vi "Set Configuration.vi"(10 "IConfigure":refnum<class "IConfigure.lvclass">, 11 "Instrument Factory in":refnum<class "Instrument Factory.lvclass">) -> (3 "Instrument Factory out":refnum<class "Instrument Factory.lvclass">)   [LabVIEW 2024, in "Instrument Factory.lvclass"]
uses:
  Interfaces/IConfigure/IConfigure.lvclass
  Instrument Factory.lvclass
  Instrument Factory.lvclass/Instrument Factory.ctl
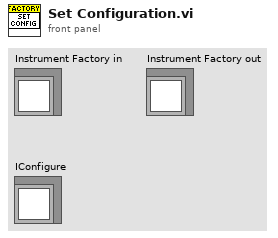
[diagram p1: front panel]
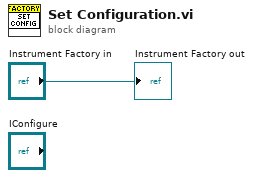
[diagram p0: block diagram]
diagram:
  "Instrument Factory out" <- "Instrument Factory in"
